vi "New Round.vi"(7 "Round":u32, 11 "MyTeam in":refnum<class "MyTeam.lvclass">) -> (3 "MyTeam out":refnum<class "MyTeam.lvclass">)   [LabVIEW 2020, in "The_Hill_Youth.lvlib" / "MyTeam.lvclass"]
doc: "This VI is called once at the beginning of each new round. This can be used to do global map updates, coordinated plans for all active squares, or nothing at all!"
uses:
  MyTeam.lvclass
  MyTeam.lvclass/MyTeam.ctl
  <vilib>/Analysis/baseanly.llb/Mean (DBL).vi
  <vilib>/Analysis/NI_AALBase.lvlib
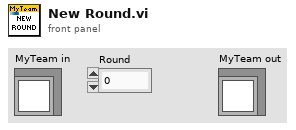
[diagram p1: front panel]
types:
  T1 = typedef "map_point.ctl" = cluster{"status":enum16{"unknown", "frind", "enemy", "empty"}, "plans":enum16{"stay", "duplicate", "attack", "move to", "no plans"}, "age":dbl}
  T2 = enum16{"stay", "duplicate", "attack", "move to", "no plans"}
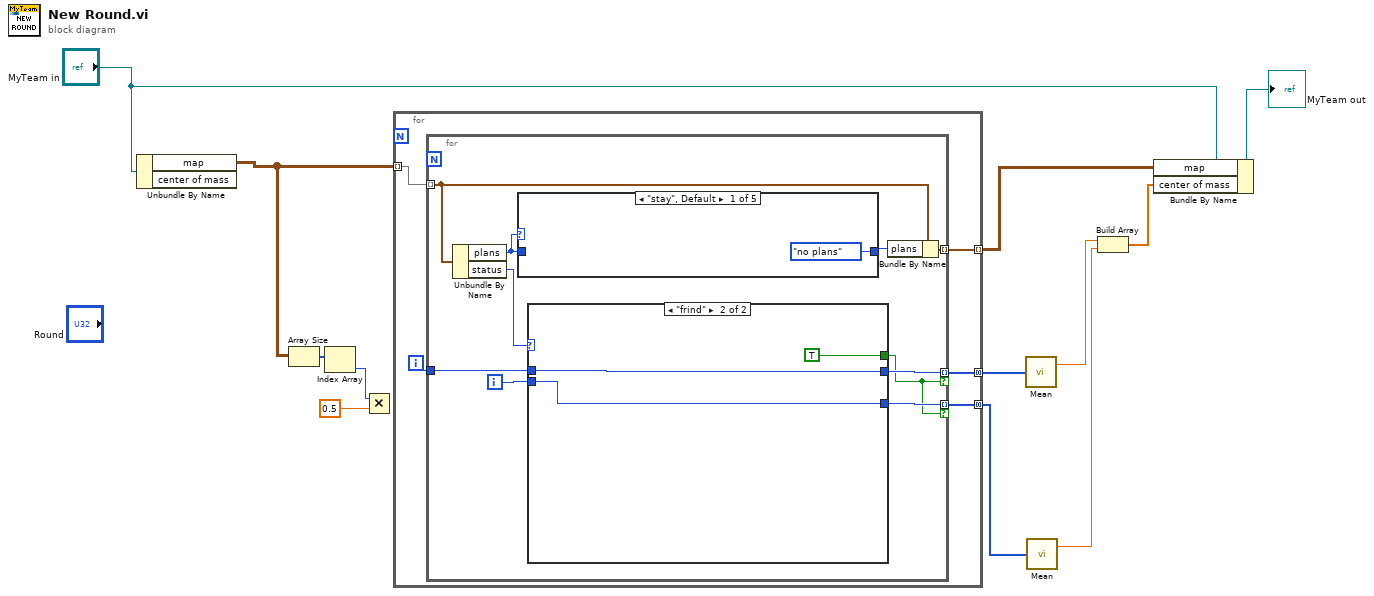
[diagram p0: block diagram]
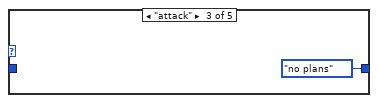
[diagram p4: hidden frame]
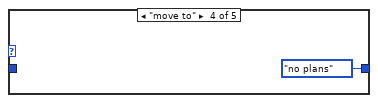
[diagram p5: hidden frame]
diagram:
  n1 = Unbundle By Name("MyTeam in") -> ("map"=w4:T1[][])  [unwired: 1 out]
  n2 = Array Size(array=w4) -> (size(s)=w3:i32[])
  n3 = Index Array(array=w3) -> (element=w1:i32)  [unwired: 1 in]
  n4 = Multiply(x=w1, y=0.5) -> ()  [unwired: 1 out]
  n5 = for {
    tunnel: w4 -> [w17] mode=indexing
    tunnel: [w16] -> w11 mode=indexing
    tunnel: [w14] -> w9 mode=concatenating
    tunnel: [w13] -> w8 mode=concatenating
    i -> [w15]
    n6 = for {
      tunnel: w17 -> [w26] mode=indexing
      tunnel: [w24] -> w16 mode=indexing
      tunnel: w15 -> [w22]
      tunnel: [w20] -> w14 mode=indexing if=w18
      tunnel: [w19] -> w13 mode=indexing if=w18
      i -> [w21]
      n7 = Unbundle By Name(w26) -> ("plans"=w27:T2, "status"=w23:enum16{"unknown", "frind", "enemy", "empty"})
      n8 = case shown="\"stay\", Default" w27 {
        tunnel: [T2."no plans" ("plans") w32 T2."no plans" ("plans") T2."no plans" ("plans") w35] -> w25
        tunnel: w27 -> [_ w32 _ _ w35]
        frame "stay", Default {
        }
        frame "duplicate" {
        }
        frame "attack" {
        }
        frame "move to" {
        }
        frame "no plans" {
        }
      }
      n9 = case shown="\"frind\"" w23 {
        tunnel: [_ TRUE] -> w18
        tunnel: w22 -> [_ w28]
        tunnel: w21 -> [_ w29]
        tunnel: [_ w28] -> w20
        tunnel: [_ w29] -> w19
        frame Default {
        }
        frame "frind" {
        }
      }
      n10 = Bundle By Name(cluster=w26, "plans"=w25) -> (w24:T1)
    }
  }
  n11 = call-poly <vilib>:"Mean.vi"("X"=w9) -> ("mean"=w7:dbl)  [unwired: 1 out]
  n12 = call-poly <vilib>:"Mean.vi"("X"=w8) -> ("mean"=w6:dbl)  [unwired: 1 out]
  n13 = Build Array(w7, w6) -> (w5:dbl[])
  n14 = Bundle By Name(cluster="MyTeam in", "map"=w11, "center of mass"=w5) -> (→"MyTeam out":refnum<class "MyTeam.lvclass">)
